vi "BackupAtTimeInterval.vi"(8 "error in (no error)":errorcluster, 11 "object in":refnum<class "TableLogger_Actor.lvclass">) -> (0 "error out":errorcluster, 3 "object out":refnum<class "TableLogger_Actor.lvclass">)   [LabVIEW 2014, in "TableLogger_Actor.lvlib" / "TableLogger_Actor.lvclass"]
uses:
  TableLogger_Actor.lvclass
  TableLogger_Actor.lvclass/TableLogger_Actor.ctl
  <vilib>/ActorFramework/Actor/Actor.lvclass/Actor.ctl
  <vilib>/ActorFramework/Message Enqueuer/Message Enqueuer.lvclass/Message Enqueuer.ctl
  <vilib>/ActorFramework/Message Enqueuer/Init from Existing Queue.vi
  <vilib>/ActorFramework/Time-Delayed Send Message/Time-Delayed Send Message.vi
  <vilib>/ActorFramework/Message Enqueuer/Message Enqueuer.lvclass
  TableLogger_Actor Messages/BackupDB Msg/BackupDB Msg.lvclass
  <vilib>/ActorFramework/Actor/Actor.lvclass
panel:
  # "Connector Pane"
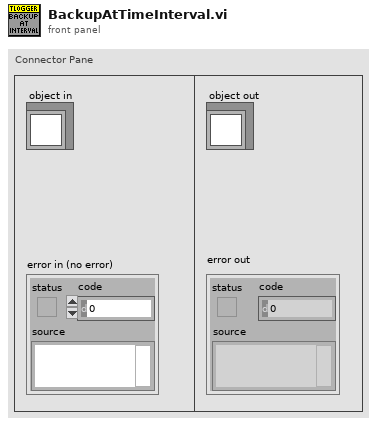
[diagram p1: front panel]
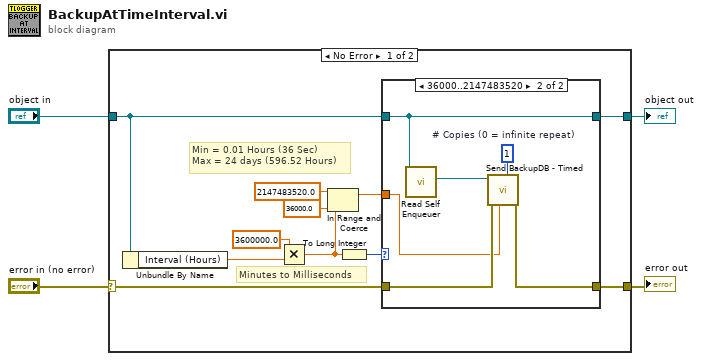
[diagram p0: block diagram]
diagram:
  n1 = case shown="No Error" "error in (no error)" {
    selector: "error in (no error)" -> [w15 w25]
    tunnel: [w13 w25] -> w2
    tunnel: [w12 w24] -> w4
    tunnel: "object in" -> [w14 w24]
    frame No Error {
      # "Min = 0.01 Hours (36 Sec)\nMax = 24 days (596.52 Hours)"
      # "Minutes to Milliseconds"
      n2 = Unbundle By Name(w14) -> ("Interval (Hours)"=w10:dbl)
      n3 = Multiply(x=3600000.0, y=w10) -> (x*y=w5:dbl)
      n4 = In Range and Coerce(upper limit=2147483520.0, x=w5, lower limit=36000.0) -> (coerced(x)=w6:dbl)  [unwired: 1 out]
      n5 = To Long Integer(number=w5) -> (32bit integer=w9:i32)
      n6 = case shown="36000..2147483520" w9 {
        tunnel: w15 -> [w17 w23]
        tunnel: [w17 w22] -> w13
        tunnel: w14 -> [w16 w19]
        tunnel: [w16 w19] -> w12
        tunnel: w6 -> [_ w18]
        frame ..0, Default {
        }
        frame 36000..2147483520 {
          w20 = u32 1  # # Copies (0 = infinite repeat)
          n7 = call <vilib>:"Read Self Enqueuer.vi"("Actor"=w19) -> ("Self Enqueuer"=w21:refnum<class "Message Enqueuer.lvclass">)  [unwired: 10 in]
          n8 = call "Send BackupDB - Timed.vi"("# Copies (0 = infinite repeat)"=w20, "Milliseconds To Wait"=w18, "error in (no error)"=w23, "Message Enqueuer"=w21) -> ("error out"=w22:errorcluster)  [unwired: 5 in, 2 out]
        }
      }
    }
    frame Error {
    }
  }
  "error out" <- w2
  "object out" <- w4
